vi "ICNC Plasma Setting Dlg.vi"(0 "HPercage":dbl, 1 "TPercage":dbl, 2 "HCoupe":dbl, 3 "Vitesse":dbl, 4 "THCVoltage":dbl, 5 "Intensite":dbl, 6 "PalpageOne":i32, 7 "error in (no error)":errorcluster caption="entrée d'erreur (pas d'erreur)", 8 "THCActif":i32, 9 "ControlePoste":i32, 10 "Simulation":i32) -> (16 "Simulation out":i32, 17 "function return":u32, 18 "THCActif out":i32, 19 "ControlePoste out":i32, 20 "HPercage out":dbl, 21 "TPercage out":dbl, 22 "HCoupe out":dbl, 23 "Vitesse out":dbl, 24 "THCVoltage out":dbl, 25 "Intensite out":dbl, 26 "PalpageOne out":i32, 27 "error out":errorcluster caption="sortie d'erreur")   [LabVIEW 2012, in "ICNC2.lvlib"]
doc: "DWORD ICNC_PlasmaSettingDlg ( double* HPercage, double* TPercage, double* HCoupe, double* Vitesse, double* THCVoltage, double* Intensite,\n int* PalpageOne, int* THCActif, int* ControlePoste, int* Simulation);"
uses:
  <userlib>/ICNC/ICNC2.lvlib
  <userlib>/ICNC/ICNC2.dll
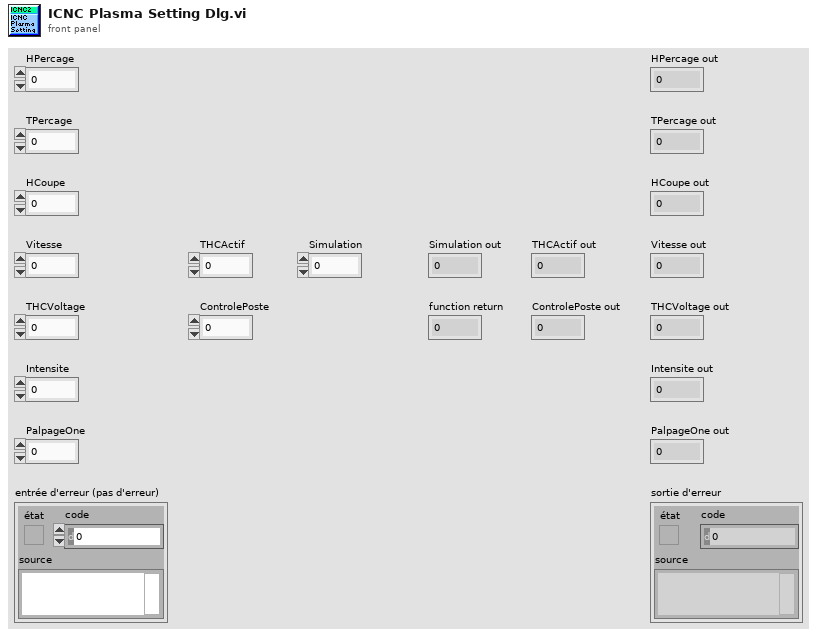
[diagram p1: front panel]
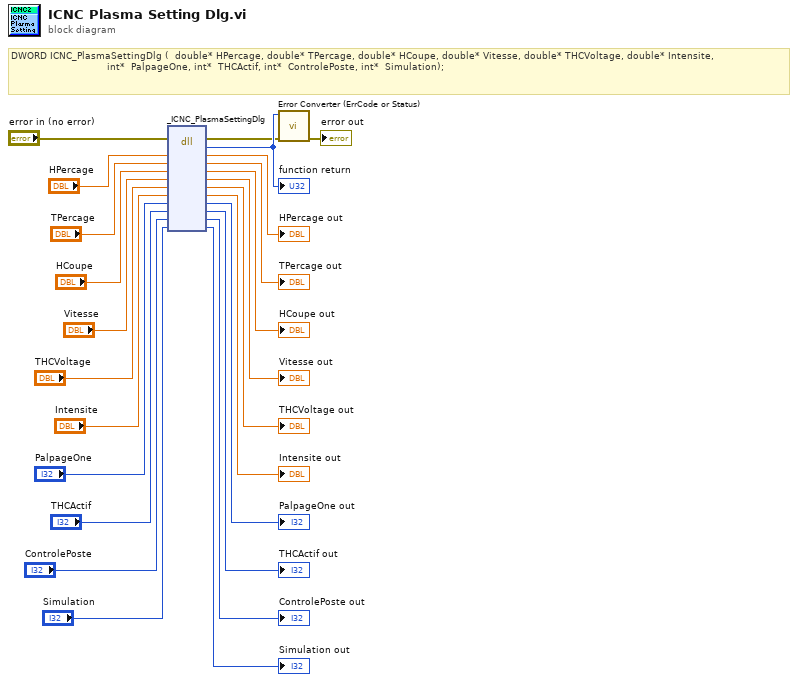
[diagram p0: block diagram]
diagram:
  # "DWORD ICNC_PlasmaSettingDlg (  double* HPercage, double* TPercage, double* HCoupe, double* Vitesse, double* THCVoltage, double* Intensite,\n                                int*  PalpageOne, int*  THCActif, int*  ControlePoste, int*  Simulation);"
  n1 = dll-call lib="C:/Program Files (x86)/National Instruments/LabVIEW 2012/user.lib/ICNC/ICNC2.*" fn="_ICNC_PlasmaSettingDlg"(error in="error in (no error)", "HPercage"="HPercage", "TPercage"="TPercage", "HCoupe"="HCoupe", "Vitesse"="Vitesse", "THCVoltage"="THCVoltage", "Intensite"="Intensite", "PalpageOne"="PalpageOne", "THCActif"="THCActif", "ControlePoste"="ControlePoste", "Simulation"="Simulation") -> (error out=w2:errorcluster, w24:u32, "HPercage"=→"HPercage out":dbl, "TPercage"=→"TPercage out":dbl, "HCoupe"=→"HCoupe out":dbl, "Vitesse"=→"Vitesse out":dbl, "THCVoltage"=→"THCVoltage out":dbl, "Intensite"=→"Intensite out":dbl, "PalpageOne"=→"PalpageOne out":i32, "THCActif"=→"THCActif out":i32, "ControlePoste"=→"ControlePoste out":i32, "Simulation"=→"Simulation out":i32)  [unwired: 2 in, 1 out]
  "function return" <- w24
  n2 = call <userlib>:"Error Converter (ErrCode or Status).vi"("error in (no error)"=w2, "error code"=w24) -> ("error out"=→"error out":errorcluster)  [unwired: 9 in]
